vi "svi_write_image_XYscan.vi"(6 "Position num":u32, 9 "chanel num":u8, 10 "image in":u16[][](array[numeric]), 11 "Chemin":path) -> ()   [LabVIEW 2013]
panel:
  out "Chaîne":string
  out "Chemin 3":path
  out "sortie d'erreur":errorcluster caption="error out"
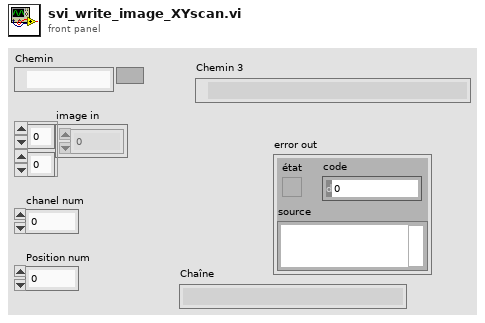
[diagram p1: front panel]
types:
  T1 = typedef "Image Type" = u32
  T2 = typedef "IMAQ Image.ctl" = refnum<image>
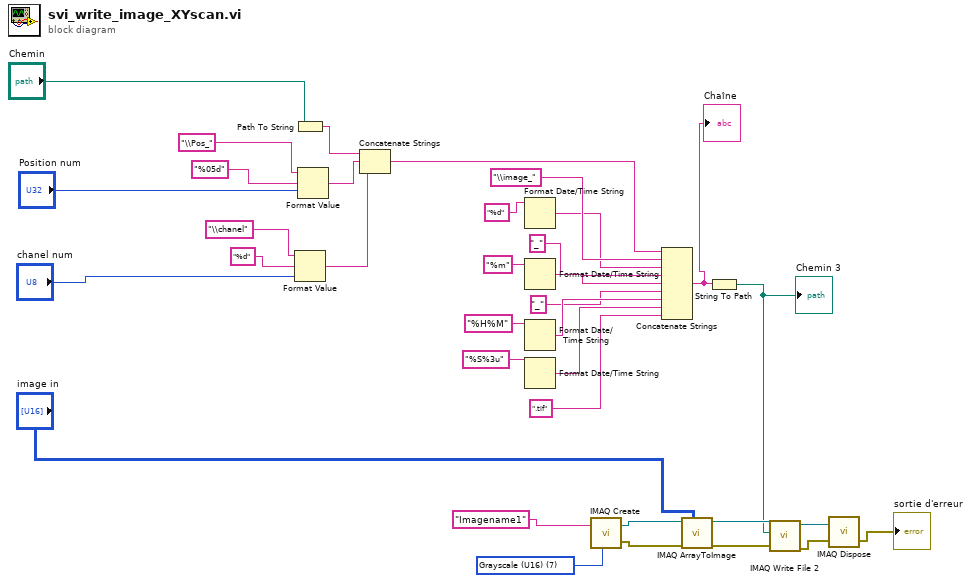
[diagram p0: block diagram]
diagram:
  w28 = T1 7 items=["Grayscale (U8)", "Grayscale (I16)", "Grayscale (SGL)", "Complex (CSG)", "RGB (U32)", "HSL (U32)", "RGB (U64)", "Grayscale (U16)"] ("Image Type")
  n1 = Path To String(path="Chemin") -> (string=w25:string)
  n2 = Format Value(string ("")="\\chanel", format string="%d" ("chaîne"), value (0)="chanel num") -> (output string=w26:string)
  n3 = Format Value(string ("")="\\Pos_", format string="%05d" ("chaîne"), value (0)="Position num") -> (output string=w2:string)
  n4 = Concatenate Strings(w25, w2, w26) -> (w3:string)
  n5 = Format Date/Time String(time format string (%c)="%d" ("chaîne")) -> (date/time string=w8:string)  [unwired: 2 out]
  n6 = Format Date/Time String(time format string (%c)="%m" ("chaîne")) -> (date/time string=w11:string)  [unwired: 2 out]
  n7 = Format Date/Time String(time format string (%c)="%H%M" ("chaîne")) -> (date/time string=w14:string)  [unwired: 2 out]
  n8 = Format Date/Time String(time format string (%c)="%S%3u" ("chaîne")) -> (date/time string=w15:string)  [unwired: 2 out]
  n9 = call "IMAQ Create"("Image Name"="Imagename1", "Image Type"=w28) -> ("New Image"=w29:T2, "error out"=w30:errorcluster)  [unwired: 2 in, 1 out]
  n10 = Concatenate Strings(w3, "\\image_", w8, "_", w11, "_", w14, w15, ".tif") -> (w1:string)
  "Chaîne" <- w1
  n11 = call "IMAQ ArrayToImage"("Image Pixels (U16)"="image in", "error in (no error)"=w30, "Image"=w29) -> ("error out"=w31:errorcluster, "Image Out"=w32:T2)  [unwired: 7 in]
  n12 = String To Path(string=w1) -> (path=w4:path)
  "Chemin 3" <- w4
  n13 = call-poly "IMAQ Write File 2"("error in (no error)"=w31, "File Path"=w4, "Image"=w32) -> ("error out"=w34:errorcluster, "Image Out (duplicate)"=w33:T2)  [unwired: 2 in, 5 out]
  n14 = call "IMAQ Dispose"("Image"=w33, "error in (no error)"=w34) -> ("error out"=→"sortie d'erreur":errorcluster)  [unwired: 1 in, 3 out]
